vi "_Remote Get Brief Status.vi"(0 "For Server? (F)":bool, 1 "error in (no error)":errorcluster) -> (2 "Status":T1 {"Corona Discharge:" format="%#.2g"; "Vac. Pressure:" format="%#.2g"; "Nebulizer Gas 2:" format="%#.2g"; "Source 2 Type:" items=["None", "ESI", "APCI", "APPI", "MicroSpray"]; "Source 1 Type:" items=["None", "ESI", "APCI", "APPI", "MicroSpray"]}, 3 "error out":errorcluster)   [LabVIEW 2015]
uses:
  Type/_Brief Status.ctl
  Type/_Source Type.ctl
  Type/_RT Command.ctl
  Type/_Log Command.ctl
  Configuration/_Global Configuration.vi
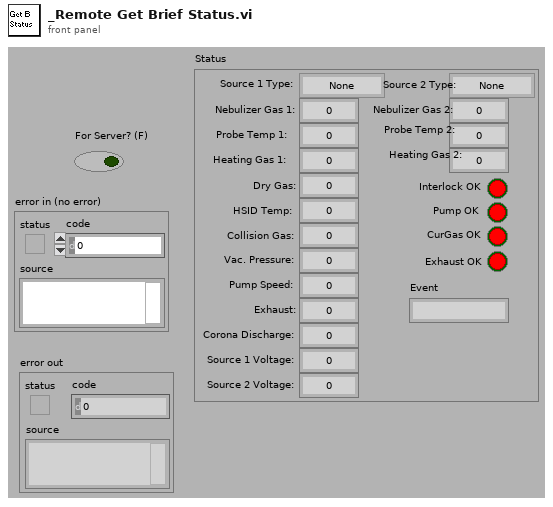
[diagram p1: front panel]
types:
  T1 = typedef "_Brief Status.ctl" = cluster{"Source 1 Type: ":T2, "Nebulizer Gas 1:":sgl, "Probe Temp 1: ":sgl, "Heating Gas 1:":sgl, "Source 2 Type:  ":T2, "Nebulizer Gas 2:":sgl, "Probe Temp 2: ":sgl, "Heating Gas 2:":sgl, "Dry Gas:":sgl, "HSID Temp:  ":sgl, "Collision Gas:":sgl, "Vac. Pressure: ":sgl, "Pump Speed:":sgl, "Exhaust:":sgl, "Interlock OK":bool, "CurGas OK":bool, "Pump OK":bool, "Exhaust OK":bool, "Event":string, "Corona Discharge:":sgl, "Source 1 Voltage:":sgl, "Source 2 Voltage:":sgl}
  T2 = typedef "_Source Type.ctl" = i8
  T3 = typedef "_RT Command.ctl" = enum16{"xml Start Run", "xml Start Actual Run", "xml Stop Run", "xml Runtime Update", "xml Get Status", "xml Get Table", "xml Set Table", "xml Get Configuration", "xml System Status", "xml Set LC Input Logic", "xml Get Data", "xml Get Info", "Start", "StartActualRun", "Stop", "Runtime Update", "Get Data", "Get Info", "Get Status", "Get Param", "Get Config", "Get Table", "Read ADC", "Set Oscillator", "Update Config", "Update Table", "Set All Pol", "Set Pol and DC", "Set Max Mass", "Toggle RP", "Toggle EL", "Set PIC", "Initialize Turbo", "Send Turbo Comm", "Close Turbo", "P1", "P2", "P3", "Send Serial", "Set LC Out", "Get LC In", "Read VAC", "Test Table", "Toggle Power", "Get Startup", "Set Startup", "Get ADC Table", "Set ADC Table", "Get Brief Status", "Get Detail Status", "Auxiliary Update", "Set CC Logics", "Set CC Input Logics", "Ignore Error", "invalid"}
  T4 = typedef "_Log Command.ctl" = enum16{"No Command", "Open", "Read", "Write", "Close", "Check Size"}
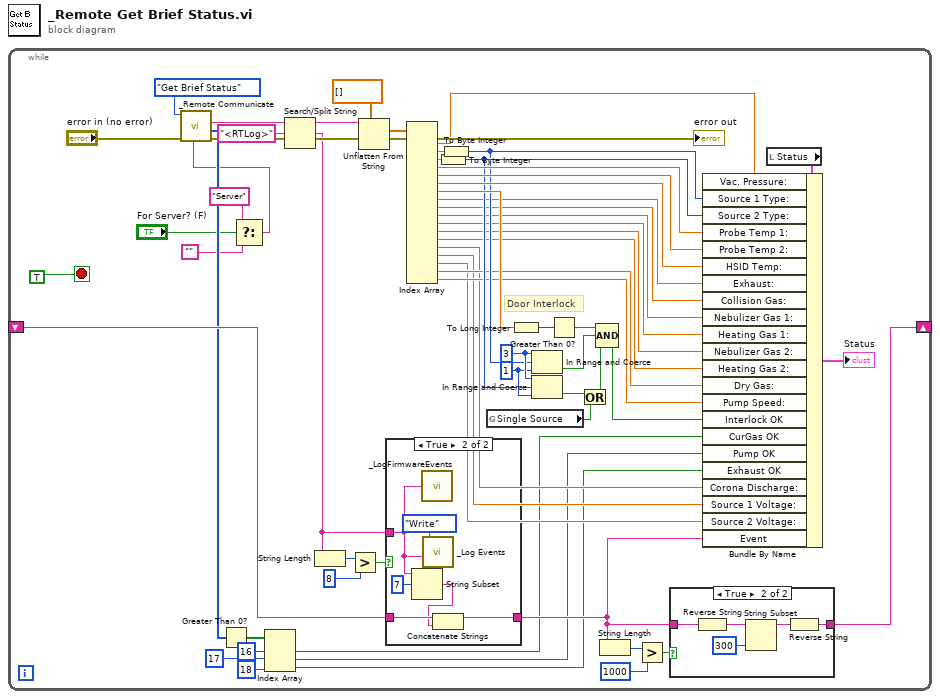
[diagram p0: block diagram]
diagram:
  n1 = while {
    shift-right: [w14] -> _
    shift-left: _ -> [w62]
    stop <- TRUE stop-if-true
    w47 = i8 1 ("lower limit")
    w48 = i8 3 ("upper limit")
    # "Door Interlock"
    n2 = Select(t="Server", s="For Server? (F)", f="") -> (s? t:f=w27:string)
    n3 = call "_Remote Communicate.vi"("String"=w27, "error in (no error)"="error in (no error)", "Command"=_RT_Command."Get Brief Status") -> ("error out"=→"error out":errorcluster, "Data Array"=w56:i32[], "Info"=w44:string)  [unwired: 3 in, 1 out]
    n4 = Greater Than 0?(x=w56) -> (x > 0?=w51:bool[])
    n5 = Index Array(array=w51, index #1=16 ("index"), index #2=17 ("index"), index #3=18 ("index")) -> (element #1=w4:bool, element #2=w3:bool, element #3=w2:bool)
    n6 = Search/Split String(string=w44, search string/char (-)="<RTLog>") -> (substring before match=w42:string, match + rest of string=w39:string)  [unwired: 2 out]
    n7 = String Length(string=w39) -> (length=w41:i32)
    n8 = Greater?(x=w41, y=8) -> (0:w38:bool)
    n9 = Unflatten From String(type=sgl[] [], binary string=w42) -> (value=w55:sgl[])  [unwired: 1 in, 4 out]
    n10 = case shown="True" w38 {
      tunnel: w39 -> [_ w70]
      tunnel: w62 -> [w69 w73]
      tunnel: [w69 w71] -> w10
      frame False {
      }
      frame True {
        n11 = String Subset(string=w70, offset (0)=7) -> (substring=w72:string)  [unwired: 1 out]
        n12 = call "_LogFirmwareEvents.vi"("Event"=w70) -> ()
        n13 = call "_Log Events.vi"("Event"=w70, "Log Command"=_Log_Command."Write" ("File Command")) -> ()  [unwired: 6 in, 2 out]
        n14 = Concatenate Strings(w73, w72) -> (w71:string)
      }
    }
    n15 = Index Array(array=w55) -> (element #1=w1:sgl, element #2=w49:sgl, element #3=w54:sgl, element #4=w33:sgl, element #5=w34:sgl, element #6=w35:sgl, element #7=w52:sgl, element #8=w25:sgl, element #9=w24:sgl, element #10=w23:sgl, element #11=w22:sgl, element #12=w21:sgl, element #13=w20:sgl, element #14=w7:sgl, element #15=w6:sgl, element #16=w5:sgl, element #17=w8:sgl, element #18=w9:sgl)  [unwired: 18 in]
    n16 = To Byte Integer(number=w54) -> (8bit integer=w32:i8)
    n17 = To Byte Integer(number=w49) -> (8bit integer=w31:i8)
    n18 = global read "_Global Configuration.vi" "Single Source"() -> (w12:bool)
    n19 = To Long Integer(number=w52) -> (32bit integer=w53:i32)
    n20 = In Range and Coerce(upper limit=w48, x=w31, lower limit=w47) -> (In Range?=w45:bool)  [unwired: 1 out]
    n21 = In Range and Coerce(upper limit=w48, x=w32, lower limit=w47) -> (In Range?=w13:bool)  [unwired: 1 out]
    n22 = Greater Than 0?(x=w53) -> (x > 0?=w46:bool)
    n23 = Or(x=w13, y=w12) -> (x .or. y?=w11:bool)
    n24 = Compound Arithmetic op=AND(w46, w45, w11) -> (w36:bool)
    n25 = String Length(string=w10) -> (length=w17:i32)
    n26 = Greater?(x=w17, y=1000) -> (0:w15:bool)
    n27 = case shown="True" w15 {
      tunnel: w10 -> [w63 w68]
      tunnel: [w63 w64] -> w14
      frame False {
      }
      frame True {
        n28 = Reverse String(1:w68) -> (0:w67:string)
        n29 = String Subset(string=w67, length (rest)=300 ("length (rest)")) -> (substring=w65:string)  [unwired: 1 out]
        n30 = Reverse String(1:w65) -> (0:w64:string)
      }
    }
    n31 = local read "Status"() -> (w37:T1)
    n32 = Bundle By Name(cluster=w37, "Vac. Pressure:"=w1, "Source 1 Type:"=w31, "Source 2 Type:"=w32, "Probe Temp 1:"=w33, "Probe Temp 2:"=w34, "HSID Temp:"=w35, "Exhaust:"=w25, "Collision Gas:"=w24, "Nebulizer Gas 1:"=w23, "Heating Gas 1:"=w22, "Nebulizer Gas 2:"=w21, "Heating Gas 2:"=w20, "Dry Gas:"=w8, "Pump Speed:"=w9, "Interlock OK"=w36, "CurGas OK"=w4, "Pump OK"=w3, "Exhaust OK"=w2, "Corona Discharge:"=w7, "Source 1 Voltage:"=w6, "Source 2 Voltage:"=w5, "Event"=w10) -> (→"Status":T1)
  }
